vi "Plot.vi"(6 "Y axis":T4, 7 "Y axis 2":T4, 8 "X axis 3":T3, 9 "X axis":T3, 10 "X axis 2":T3, 11 "Measurement Arrays":T1) -> (0 "MOKE X,Y":T2(array[cluster]), 2 "MOKE 2":T5, 3 "MOKE":T6)   [LabVIEW 2017]
uses:
  Yaxis.ctl
  Xaxis.ctl
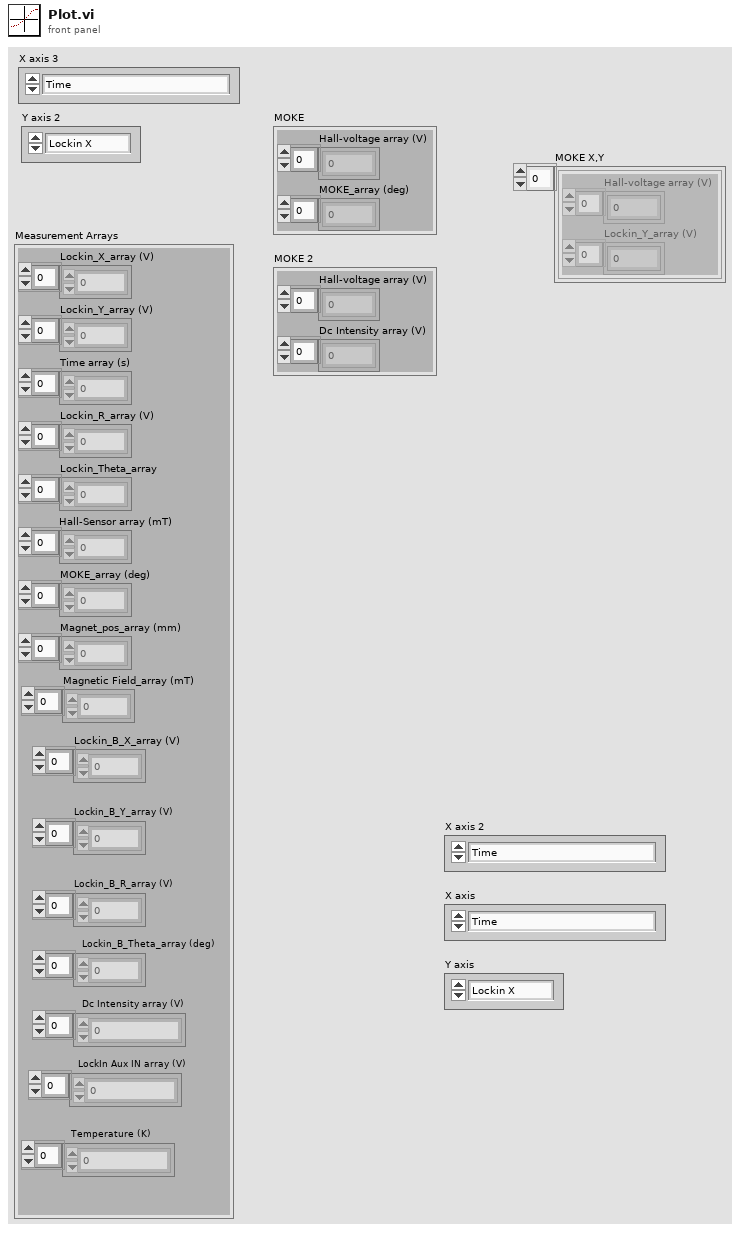
[diagram p1: front panel]
types:
  T1 = cluster{"Lockin_X_array (V)":dbl[], "Lockin_Y_array (V)":dbl[], "Time array (s)":dbl[], "Lockin_R_array (V)":dbl[], "Lockin_Theta_array":dbl[], "Hall-Sensor array (mT)":dbl[], "MOKE_array (deg)":dbl[], "Magnet_pos_array (mm)":dbl[], "Magnetic Field_array (mT)":dbl[], "Lockin_B_X_array (V)":dbl[], "Lockin_B_Y_array (V)":dbl[], "Lockin_B_R_array (V)":dbl[], "Lockin_B_Theta_array (deg)":dbl[], "Dc Intensity array (V)":dbl[], "LockIn Aux IN array (V)":dbl[], "Temperature (K)":dbl[]}
  T2 = cluster{"Hall-voltage array (V)":dbl[], "Lockin_Y_array (V)":dbl[]}[]
  T3 = typedef "Xaxis.ctl" = enum16{"Time", "Magnetic Field", "Magnet Position", "Hall Sensor"}
  T4 = typedef "Yaxis.ctl" = enum16{"Lockin X", "Lockin Y", "Lockin R", "Lockin Theta", "MOKE (deg)", "Dc Intensity (V)"}
  T5 = cluster{"Hall-voltage array (V)":dbl[], "Dc Intensity array (V)":dbl[]}
  T6 = cluster{"Hall-voltage array (V)":dbl[], "MOKE_array (deg)":dbl[]}
  T7 = cluster{"Hall-Sensor array (mT)":dbl[], "LockIn Aux IN array (V)":dbl[]}
  T8 = cluster{"Hall-Sensor array (mT)":dbl[], "MOKE_array (deg)":dbl[]}
  T9 = cluster{"Hall-Sensor array (mT)":dbl[], "Lockin_Y_array (V)":dbl[]}
  T10 = cluster{"Hall-Sensor array (mT)":dbl[], "Lockin_X_array (V)":dbl[]}
  T11 = cluster{"Hall-Sensor array (mT)":dbl[], "Lockin_Y_array (V)":dbl[]}[]
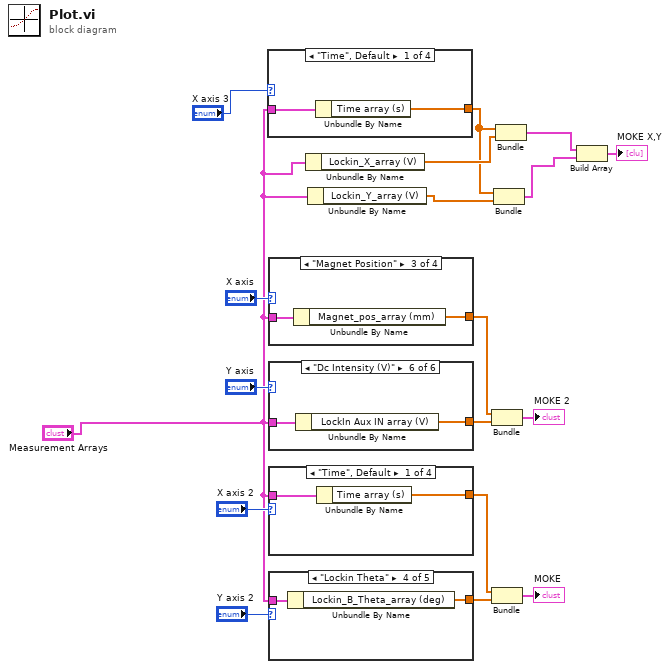
[diagram p0: block diagram]
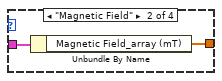
[diagram p2: hidden frame]
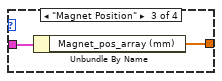
[diagram p3: hidden frame]
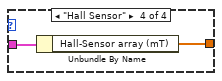
[diagram p4: hidden frame]
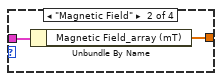
[diagram p5: hidden frame]
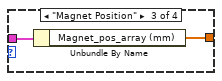
[diagram p6: hidden frame]
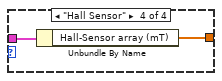
[diagram p7: hidden frame]
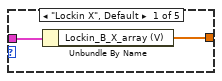
[diagram p8: hidden frame]
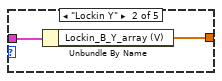
[diagram p9: hidden frame]
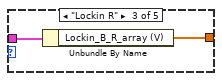
[diagram p10: hidden frame]
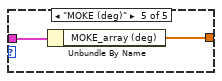
[diagram p11: hidden frame]
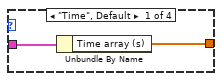
[diagram p12: hidden frame]
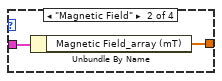
[diagram p13: hidden frame]
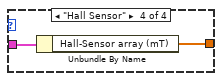
[diagram p14: hidden frame]
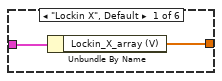
[diagram p15: hidden frame]
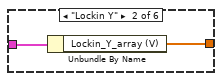
[diagram p16: hidden frame]
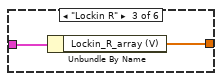
[diagram p17: hidden frame]
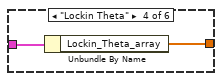
[diagram p18: hidden frame]
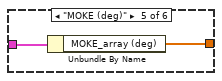
[diagram p19: hidden frame]
diagram:
  n1 = case shown="\"Time\", Default" "X axis 3" {
    tunnel: [w20 w22 w24 w25] -> w6
    tunnel: "Measurement Arrays" -> [w19 w21 w23 w26]
    frame "Time", Default {
      n2 = Unbundle By Name(w19) -> ("Time array (s)"=w20:dbl[])
    }
    frame "Magnetic Field" {
      n3 = Unbundle By Name(w21) -> ("Magnetic Field_array (mT)"=w22:dbl[])
    }
    frame "Magnet Position" {
      n4 = Unbundle By Name(w23) -> ("Magnet_pos_array (mm)"=w24:dbl[])
    }
    frame "Hall Sensor" {
      n5 = Unbundle By Name(w26) -> ("Hall-Sensor array (mT)"=w25:dbl[])
    }
  }
  n6 = case shown="\"Magnet Position\"" "X axis" {
    tunnel: [w28 w30 w32 w33] -> w9
    tunnel: "Measurement Arrays" -> [w27 w29 w31 w34]
    frame "Time", Default {
      n7 = Unbundle By Name(w27) -> ("Time array (s)"=w28:dbl[])
    }
    frame "Magnetic Field" {
      n8 = Unbundle By Name(w29) -> ("Magnetic Field_array (mT)"=w30:dbl[])
    }
    frame "Magnet Position" {
      n9 = Unbundle By Name(w31) -> ("Magnet_pos_array (mm)"=w32:dbl[])
    }
    frame "Hall Sensor" {
      n10 = Unbundle By Name(w34) -> ("Hall-Sensor array (mT)"=w33:dbl[])
    }
  }
  n11 = case shown="\"Dc Intensity (V)\"" "Y axis" {
    tunnel: [w36 w38 w40 w42 w44 w45] -> w10
    tunnel: "Measurement Arrays" -> [w35 w37 w39 w41 w43 w46]
    frame "Lockin X", Default {
      n12 = Unbundle By Name(w35) -> ("Lockin_X_array (V)"=w36:dbl[])
    }
    frame "Lockin Y" {
      n13 = Unbundle By Name(w37) -> ("Lockin_Y_array (V)"=w38:dbl[])
    }
    frame "Lockin R" {
      n14 = Unbundle By Name(w39) -> ("Lockin_R_array (V)"=w40:dbl[])
    }
    frame "Lockin Theta" {
      n15 = Unbundle By Name(w41) -> ("Lockin_Theta_array"=w42:dbl[])
    }
    frame "MOKE (deg)" {
      n16 = Unbundle By Name(w43) -> ("MOKE_array (deg)"=w44:dbl[])
    }
    frame "Dc Intensity (V)" {
      n17 = Unbundle By Name(w46) -> ("LockIn Aux IN array (V)"=w45:dbl[])
    }
  }
  n18 = case shown="\"Time\", Default" "X axis 2" {
    tunnel: [w48 w50 w52 w54] -> w15
    tunnel: "Measurement Arrays" -> [w47 w49 w51 w53]
    frame "Time", Default {
      n19 = Unbundle By Name(w47) -> ("Time array (s)"=w48:dbl[])
    }
    frame "Magnetic Field" {
      n20 = Unbundle By Name(w49) -> ("Magnetic Field_array (mT)"=w50:dbl[])
    }
    frame "Magnet Position" {
      n21 = Unbundle By Name(w51) -> ("Magnet_pos_array (mm)"=w52:dbl[])
    }
    frame "Hall Sensor" {
      n22 = Unbundle By Name(w53) -> ("Hall-Sensor array (mT)"=w54:dbl[])
    }
  }
  n23 = case shown="\"Lockin Theta\"" "Y axis 2" {
    tunnel: [w56 w58 w60 w62 w64] -> w14
    tunnel: "Measurement Arrays" -> [w55 w57 w59 w61 w63]
    frame "Lockin X", Default {
      n24 = Unbundle By Name(w55) -> ("Lockin_B_X_array (V)"=w56:dbl[])
    }
    frame "Lockin Y" {
      n25 = Unbundle By Name(w57) -> ("Lockin_B_Y_array (V)"=w58:dbl[])
    }
    frame "Lockin R" {
      n26 = Unbundle By Name(w59) -> ("Lockin_B_R_array (V)"=w60:dbl[])
    }
    frame "Lockin Theta" {
      n27 = Unbundle By Name(w61) -> ("Lockin_B_Theta_array (deg)"=w62:dbl[])
    }
    frame "MOKE (deg)" {
      n28 = Unbundle By Name(w63) -> ("MOKE_array (deg)"=w64:dbl[])
    }
  }
  n29 = Unbundle By Name("Measurement Arrays") -> ("Lockin_X_array (V)"=w7:dbl[])
  n30 = Unbundle By Name("Measurement Arrays") -> ("Lockin_Y_array (V)"=w5:dbl[])
  n31 = Bundle("Hall-Sensor array (mT)"=w9, "LockIn Aux IN array (V)"=w10) -> (→"MOKE 2":T7)  [unwired: 1 in]
  n32 = Bundle("Hall-Sensor array (mT)"=w15, "MOKE_array (deg)"=w14) -> (→"MOKE":T8)  [unwired: 1 in]
  n33 = Bundle("Hall-Sensor array (mT)"=w6, "Lockin_Y_array (V)"=w5) -> (w3:T9)  [unwired: 1 in]
  n34 = Bundle("Hall-Sensor array (mT)"=w6, "Lockin_X_array (V)"=w7) -> (w4:T10)  [unwired: 1 in]
  n35 = Build Array(w4, w3) -> (→"MOKE X,Y":T11)
